vi "Lab Panel V5.22.1.vi"() -> ()   [LabVIEW 2013] (continued)
                            n2498 = Bundle(cluster=w4642, "amps"=w4646, "volts"=w4645, "pf"=w4644) -> (w4643:cluster{"amps":dbl, "volts":dbl, "pf":dbl})
                            n2499 = local write "ON L05-2"(w4643) -> ()
                          }
                        }
                      }
                      frame #1 {
                        n2500 = Unbundle(w4651) -> ("amps"=w4650:dbl, "volts"=w4649:dbl, "pf"=w4648:dbl)
                        n2501 = case shown="True" w4652 {
                          tunnel: w4659 -> [_ w4691]
                          tunnel: w4658 -> [_ w4698]
                          tunnel: w4657 -> [_ _]
                          tunnel: w4656 -> [_ _]
                          tunnel: w4655 -> [_ w4697]
                          tunnel: w4654 -> [_ w4696]
                          tunnel: w4653 -> [_ w4661]
                          tunnel: w4650 -> [_ w4693]
                          tunnel: w4649 -> [_ w4692]
                          tunnel: w4648 -> [_ w4690]
                          tunnel: w4647 -> [_ w4682]
                          frame False {
                          }
                          frame True {
                            n2502 = local read "TDMS LAB05-2"() -> (w4695:refnum<k34>)
                            n2503 = Build Array(w4692) -> (w4687:dbl[])
                            n2504 = Build Array(w4690) -> (w4686:dbl[])
                            n2505 = Build Array(w4697) -> (w4685:dbl[])
                            n2506 = Build Array(w4698) -> (w4684:dbl[])
                            n2507 = Build Array(w4693) -> (w4689:dbl[])
                            n2508 = Build Array(w4691) -> (w4688:dbl[])
                            n2509 = Build Array(w4696) -> (w4683:dbl[])
                            n2510 = Build Array("AMPS ON", "AMPS OFF", "VOLTS", "PF", "TEMP Live", "TEMP Neut", "CYCLE") -> (w4666:string[])
                            n2511 = Bundle By Name("Y"=w4689, "t0"=w4682) -> (w4681:waveform(dbl))  [unwired: 1 in]
                            n2512 = Bundle By Name("Y"=w4688, "t0"=w4682) -> (w4680:waveform(dbl))  [unwired: 1 in]
                            n2513 = Bundle By Name("Y"=w4687, "t0"=w4682) -> (w4679:waveform(dbl))  [unwired: 1 in]
                            n2514 = Bundle By Name("Y"=w4686, "t0"=w4682) -> (w4678:waveform(dbl))  [unwired: 1 in]
                            n2515 = Bundle By Name("Y"=w4685, "t0"=w4682) -> (w4677:waveform(dbl))  [unwired: 1 in]
                            n2516 = Bundle By Name("Y"=w4684, "t0"=w4682) -> (w4676:waveform(dbl))  [unwired: 1 in]
                            n2517 = Bundle By Name("Y"=w4683, "t0"=w4682) -> (w4675:waveform(dbl))  [unwired: 1 in]
                            n2518 = Build Array(w4681, w4680, w4679, w4678, w4677, w4676, w4675) -> (w4674:waveform(dbl)[])
                            n2519 = TDMS Write(0:w4695, 5:"TEST VALUES", 7:w4666, 9:w4674) -> (4:w4665:refnum<k34>, 6:w4664:string, 15:w4663:errorcluster)  [unwired: 2 in, 1 out]
                            n2520 = TDMS Write(0:w4665, 5:w4664, 7:"TIME", 9:w4661, 11:w4663) -> (15:w4660:errorcluster)  [unwired: 1 in, 3 out]
                            n2521 = local write "data file error"(w4660) -> ()
                          }
                        }
                      }
                    }
                  }
                }
              }
            }
          }
          frame #13 {
            # "display test values on chart"
            n2522 = local read "jig cycle"() -> (w4703:dbl)
            n2523 = local read "on loops"() -> (w4705:dbl)
            n2524 = Add(x=w4705, y=2) -> (x+y=w4702:dbl)
            n2525 = Equal?(x=w4703, y=1) -> (x = y?=w4701:bool)
            n2526 = Equal?(x=w4703, y=w4702) -> (x = y?=w4700:bool)
            n2527 = Or(x=w4701, y=w4700) -> (x .or. y?=w4699:bool)
            "graph flag" <- w4699
            n2528 = global write "Global display 3.vi" "graph flag"(w4699) -> ()
            n2529 = case shown="True" w4699 {
              frame False {
              }
              frame True {
                n2530 = local read "SIG LAB05-1"() -> (w4748:T2)
                n2531 = local read "SIG LAB04-2"() -> (w4749:T2)
                n2532 = local read "SIG LAB05-2"() -> (w4747:T2)
                n2533 = local read "SIG LAB04-1"() -> (w4750:T2)
                n2534 = local read "SIG LAB03-1"() -> (w4752:T2)
                n2535 = local read "SIG LAB03-2"() -> (w4751:T2)
                n2536 = local read "SIG LAB01-1"() -> (w4756:T2)
                n2537 = local read "SIG LAB02-2"() -> (w4753:T2)
                n2538 = local read "SIG LAB02-1"() -> (w4754:T2)
                n2539 = local read "SIG LAB01-2"() -> (w4755:T2)
                n2540 = Unbundle(w4749) -> ("AMPS"=w4739:dbl, "VOLTS"=w4729:dbl, "Tmp Live"=w4719:dbl, "Tmp Neut"=w4709:dbl)  [unwired: 1 out]
                n2541 = Unbundle(w4748) -> ("AMPS"=w4738:dbl, "VOLTS"=w4728:dbl, "Tmp Live"=w4718:dbl, "Tmp Neut"=w4708:dbl)  [unwired: 1 out]
                n2542 = Unbundle(w4747) -> ("AMPS"=w4737:dbl, "VOLTS"=w4727:dbl, "Tmp Live"=w4717:dbl, "Tmp Neut"=w4707:dbl)  [unwired: 1 out]
                n2543 = Unbundle(w4750) -> ("AMPS"=w4740:dbl, "VOLTS"=w4730:dbl, "Tmp Live"=w4720:dbl, "Tmp Neut"=w4710:dbl)  [unwired: 1 out]
                n2544 = Unbundle(w4751) -> ("AMPS"=w4741:dbl, "VOLTS"=w4731:dbl, "Tmp Live"=w4721:dbl, "Tmp Neut"=w4711:dbl)  [unwired: 1 out]
                n2545 = Unbundle(w4752) -> ("AMPS"=w4742:dbl, "VOLTS"=w4732:dbl, "Tmp Live"=w4722:dbl, "Tmp Neut"=w4712:dbl)  [unwired: 1 out]
                n2546 = Unbundle(w4753) -> ("AMPS"=w4743:dbl, "VOLTS"=w4733:dbl, "Tmp Live"=w4723:dbl, "Tmp Neut"=w4713:dbl)  [unwired: 1 out]
                n2547 = Unbundle(w4754) -> ("AMPS"=w4744:dbl, "VOLTS"=w4734:dbl, "Tmp Live"=w4724:dbl, "Tmp Neut"=w4714:dbl)  [unwired: 1 out]
                n2548 = Unbundle(w4756) -> ("AMPS"=w4746:dbl, "VOLTS"=w4736:dbl, "Tmp Live"=w4726:dbl, "Tmp Neut"=w4716:dbl)  [unwired: 1 out]
                n2549 = Unbundle(w4755) -> ("AMPS"=w4745:dbl, "VOLTS"=w4735:dbl, "Tmp Live"=w4725:dbl, "Tmp Neut"=w4715:dbl)  [unwired: 1 out]
                n2550 = stacked-sequence {
                  tunnel: w4746 -> [w4788 _ _]
                  tunnel: w4745 -> [w4787 _ _]
                  tunnel: w4744 -> [w4778 _ _]
                  tunnel: w4743 -> [w4777 _ _]
                  tunnel: w4742 -> [w4767 _ _]
                  tunnel: w4741 -> [w4766 _ _]
                  tunnel: w4740 -> [_ w4811 _]
                  tunnel: w4739 -> [_ w4810 _]
                  tunnel: w4738 -> [_ w4800 _]
                  tunnel: w4737 -> [_ w4799 _]
                  tunnel: w4736 -> [w4785 _ _]
                  tunnel: w4735 -> [w4784 _ _]
                  tunnel: w4734 -> [w4775 _ _]
                  tunnel: w4733 -> [w4774 _ _]
                  tunnel: w4732 -> [w4765 _ _]
                  tunnel: w4731 -> [w4764 _ _]
                  tunnel: w4730 -> [_ w4809 _]
                  tunnel: w4729 -> [_ w4808 _]
                  tunnel: w4728 -> [_ w4798 _]
                  tunnel: w4727 -> [_ w4797 _]
                  tunnel: w4726 -> [w4782 _ _]
                  tunnel: w4725 -> [w4780 _ _]
                  tunnel: w4724 -> [w4771 _ _]
                  tunnel: w4723 -> [w4769 _ _]
                  tunnel: w4722 -> [w4763 _ _]
                  tunnel: w4721 -> [w4761 _ _]
                  tunnel: w4720 -> [_ w4807 _]
                  tunnel: w4719 -> [_ w4805 _]
                  tunnel: w4718 -> [_ w4796 _]
                  tunnel: w4717 -> [_ w4794 _]
                  tunnel: w4716 -> [w4781 _ _]
                  tunnel: w4715 -> [w4779 _ _]
                  tunnel: w4714 -> [w4770 _ _]
                  tunnel: w4713 -> [w4768 _ _]
                  tunnel: w4712 -> [w4762 _ _]
                  tunnel: w4711 -> [w4760 _ _]
                  tunnel: w4710 -> [_ w4806 _]
                  tunnel: w4709 -> [_ w4804 _]
                  tunnel: w4708 -> [_ w4795 _]
                  tunnel: w4707 -> [_ w4793 _]
                  frame #0 {
                    n2551 = Merge Signals(w4788, w4787) -> (→"LAB01 AMPS":dynamicdata)
                    n2552 = Merge Signals(w4785, w4784) -> (→"LAB01 VOLTS":dynamicdata)
                    n2553 = Merge Signals(w4765, w4764) -> (→"LAB03 VOLTS":dynamicdata)
                    n2554 = Merge Signals(w4782, w4781, w4780, w4779) -> (→"LAB01 deg C":dynamicdata)
                    n2555 = Merge Signals(w4778, w4777) -> (→"LAB02 AMPS":dynamicdata)
                    n2556 = Merge Signals(w4771, w4770, w4769, w4768) -> (→"LAB02 deg C":dynamicdata)
                    n2557 = Merge Signals(w4763, w4762, w4761, w4760) -> (→"LAB03 deg C":dynamicdata)
                    n2558 = Merge Signals(w4775, w4774) -> (→"LAB02 VOLTS":dynamicdata)
                    n2559 = Merge Signals(w4767, w4766) -> (→"LAB03 AMPS":dynamicdata)
                  }
                  frame #1 {
                    n2560 = Merge Signals(w4798, w4797) -> (→"LAB05 VOLTS":dynamicdata)
                    n2561 = Merge Signals(w4811, w4810) -> (→"LAB04 AMPS":dynamicdata)
                    n2562 = Merge Signals(w4800, w4799) -> (→"LAB05 AMPS":dynamicdata)
                    n2563 = Merge Signals(w4796, w4795, w4794, w4793) -> (→"LAB05 deg C":dynamicdata)
                    n2564 = Merge Signals(w4807, w4806, w4805, w4804) -> (→"LAB04 deg C":dynamicdata)
                    n2565 = Merge Signals(w4809, w4808) -> (→"LAB04 VOLTS":dynamicdata)
                  }
                  frame #2 {
                    n2566 = local read "LAB05 VOLTS"() -> (w4819:dynamicdata)
                    n2567 = local read "LAB04 VOLTS"() -> (w4820:dynamicdata)
                    n2568 = local read "LAB02 VOLTS"() -> (w4822:dynamicdata)
                    n2569 = local read "LAB03 VOLTS"() -> (w4821:dynamicdata)
                    n2570 = local read "LAB05 AMPS"() -> (w4825:dynamicdata)
                    n2571 = local read "LAB01 VOLTS"() -> (w4823:dynamicdata)
                    n2572 = local read "LAB04 AMPS"() -> (w4826:dynamicdata)
                    n2573 = local read "LAB03 AMPS"() -> (w4827:dynamicdata)
                    n2574 = local read "LAB03 deg C"() -> (w4815:dynamicdata)
                    n2575 = local read "LAB02 AMPS"() -> (w4828:dynamicdata)
                    n2576 = local read "LAB04 deg C"() -> (w4814:dynamicdata)
                    n2577 = local read "LAB05 deg C"() -> (w4813:dynamicdata)
                    n2578 = local read "LAB02 deg C"() -> (w4816:dynamicdata)
                    n2579 = local read "LAB01 deg C"() -> (w4817:dynamicdata)
                    n2580 = local read "LAB01 AMPS"() -> (w4829:dynamicdata)
                    n2581 = Merge Signals(w4817, w4816, w4815, w4814, w4813) -> (w4812:dynamicdata)
                    n2582 = Merge Signals(w4829, w4828, w4827, w4826, w4825) -> (w4824:dynamicdata)
                    n2583 = Merge Signals(w4823, w4822, w4821, w4820, w4819) -> (w4818:dynamicdata)
                    n2584 = global write "Global display 3.vi" "graph volts"(w4818) -> ()
                    n2585 = global write "Global display 3.vi" "graph deg C"(w4812) -> ()
                    n2586 = global write "Global display 3.vi" "graph amps"(w4824) -> ()
                  }
                }
              }
            }
          }
          frame #14 {
            # "check for amps fail"
            # "check for cycle test & temperature rise fail conditions"
            n2587 = local read "on loops"() -> (w4856:dbl)
            n2588 = local read "jig cycle"() -> (w4853:dbl)
            n2589 = local read "jig cycle"() -> (w4858:dbl)
            n2590 = Add(x=w4856, y=3.0) -> (x+y=w4854:dbl)
            n2591 = Equal?(x=w4853, y=w4854) -> (x = y?=w4849:bool)
            n2592 = local read "Fail Loops"() -> (w4830:dbl)
            n2593 = Equal?(x=w4858, y=1.0) -> (x = y?=w4851:bool)
            n2594 = global write "Global 1.vi" "fail count"(w4830) -> ()
            n2595 = stacked-sequence {
              tunnel: w4852 -> [w4861 _ _ _ _ _ _ _ _ _]
              tunnel: w4851 -> [w4862 w4882 w4902 w4922 w4942 w4962 w4982 w5002 w5022 w5042]
              tunnel: w4850 -> [w4859 _ _ _ _ _ _ _ _ _]
              tunnel: w4849 -> [w4860 w4881 w4901 w4921 w4941 w4961 w4981 w5001 w5021 w5041]
              tunnel: w4848 -> [_ w4880 _ _ _ _ _ _ _ _]
              tunnel: w4847 -> [_ w4879 _ _ _ _ _ _ _ _]
              tunnel: w4846 -> [_ _ w4900 _ _ _ _ _ _ _]
              tunnel: w4845 -> [_ _ w4899 _ _ _ _ _ _ _]
              tunnel: w4844 -> [_ _ _ w4920 _ _ _ _ _ _]
              tunnel: w4843 -> [_ _ _ w4919 _ _ _ _ _ _]
              tunnel: w4842 -> [_ _ _ _ w4940 _ _ _ _ _]
              tunnel: w4841 -> [_ _ _ _ w4939 _ _ _ _ _]
              tunnel: w4840 -> [_ _ _ _ _ w4960 _ _ _ _]
              tunnel: w4839 -> [_ _ _ _ _ w4959 _ _ _ _]
              tunnel: w4838 -> [_ _ _ _ _ _ w4980 _ _ _]
              tunnel: w4837 -> [_ _ _ _ _ _ w4979 _ _ _]
              tunnel: w4836 -> [_ _ _ _ _ _ _ w5000 _ _]
              tunnel: w4835 -> [_ _ _ _ _ _ _ w4999 _ _]
              tunnel: w4834 -> [_ _ _ _ _ _ _ _ w5020 _]
              tunnel: w4833 -> [_ _ _ _ _ _ _ _ w5019 _]
              tunnel: w4832 -> [_ _ _ _ _ _ _ _ _ w5040]
              tunnel: w4831 -> [_ _ _ _ _ _ _ _ _ w5039]
              frame #0 {
                # "LAB01-1"
                n2596 = case shown="True" w4859 {
                  tunnel: w4862 -> [_ w4875]
                  tunnel: w4861 -> [_ w4872]
                  tunnel: w4860 -> [_ w4871]
                  frame False {
                  }
                  frame True {
                    n2597 = local read "TEMP START LAB01-1"() -> (w4877:cluster{"TL":dbl, "TN":dbl})
                    n2598 = local read "RESULT LAB01-1"() -> (w4866:bool)
                    n2599 = local read "FAIL LAB01-1"() -> (w4869:cluster{"LO":dbl, "HI":dbl})
                    n2600 = local read "TDMS LAB01-1"() -> (w4876:refnum<k34>)
                    n2601 = local read "SET LAB01-1"() -> (w4873:T5)
                    n2602 = local read "DISP LAB01-1"() -> (w4874:T4)
                    n2603 = local read "SIG LAB01-1"() -> (w4878:T2)
                    n2604 = Bundle("FAIL LAB01-1"=w4869, "SIG LAB01-1"=w4878, "TEMP START LAB01-1"=w4877, "DISP LAB01-1"=w4874, "SET LAB01-1"=w4873, "TDMS LAB01-1"=w4876) -> (w4863:T33)  [unwired: 1 in]
                    n2605 = call "sub vi - cycle&temp fail v7.vi"("Amps Lo?"=w4875, "Input Cluster"=w4863, "SELECT"=w4872, "Amps Hi?"=w4871, "Result In"=w4866) -> ("(FAIL) out"=w4868:cluster{"FAIL LO":dbl, "FAIL HI":dbl}, "(DISP) out"=w4864:T4, "T-RISE"=w4865:cluster{"T-RISE (L)":dbl, "T-RISE (N)":dbl}, "Result Out"=w4867:bool, "file error"=w4870:errorcluster)  [unwired: 10 in]
                    n2606 = local write "TEMP RISE LAB01-1"(w4865) -> ()
                    n2607 = local write "FAIL LAB01-1"(w4868) -> ()
                    n2608 = local write "DISP LAB01-1"(w4864) -> ()
                    n2609 = local write "RESULT LAB01-1"(w4867) -> ()
                    n2610 = local write "data file error"(w4870) -> ()
                  }
                }
              }
              frame #1 {
                # "LAB01-2"
                n2611 = case shown="True" w4880 {
                  tunnel: w4882 -> [_ w4895]
                  tunnel: w4879 -> [_ w4892]
                  tunnel: w4881 -> [_ w4891]
                  frame False {
                  }
                  frame True {
                    n2612 = local read "TEMP START LAB01-2"() -> (w4897:cluster{"TL":dbl, "TN":dbl})
                    n2613 = local read "FAIL LAB01-2"() -> (w4888:cluster{"LO":dbl, "HI":dbl})
                    n2614 = local read "TDMS LAB01-2"() -> (w4896:refnum<k34>)
                    n2615 = local read "SET LAB01-2"() -> (w4893:T5)
                    n2616 = local read "DISP LAB01-2"() -> (w4894:T4)
                    n2617 = local read "RESULT LAB01-2"() -> (w4885:bool)
                    n2618 = local read "SIG LAB01-2"() -> (w4898:T2)
                    n2619 = Bundle("FAIL LAB01-2"=w4888, "SIG LAB01-2"=w4898, "TEMP START LAB01-2"=w4897, "DISP LAB01-2"=w4894, "SET LAB01-2"=w4893, "TDMS LAB01-2"=w4896) -> (w4883:T34)  [unwired: 1 in]
                    n2620 = call "sub vi - cycle&temp fail v7.vi"("Amps Lo?"=w4895, "Input Cluster"=w4883, "SELECT"=w4892, "Amps Hi?"=w4891, "Result In"=w4885) -> ("(FAIL) out"=w4887:cluster{"FAIL LO":dbl, "FAIL HI":dbl}, "(DISP) out"=w4890:T4, "T-RISE"=w4884:cluster{"T-RISE (L)":dbl, "T-RISE (N)":dbl}, "Result Out"=w4886:bool, "file error"=w4889:errorcluster)  [unwired: 10 in]
                    n2621 = local write "TEMP RISE LAB01-2"(w4884) -> ()
                    n2622 = local write "FAIL LAB01-2"(w4887) -> ()
                    n2623 = local write "DISP LAB01-2"(w4890) -> ()
                    n2624 = local write "RESULT LAB01-2"(w4886) -> ()
                    n2625 = local write "data file error"(w4889) -> ()
                  }
                }
              }
              frame #2 {
                # "LAB02-1"
                n2626 = case shown="True" w4900 {
                  tunnel: w4902 -> [_ w4915]
                  tunnel: w4899 -> [_ w4912]
                  tunnel: w4901 -> [_ w4911]
                  frame False {
                  }
                  frame True {
                    n2627 = local read "TEMP START LAB02-1"() -> (w4917:cluster{"TL":dbl, "TN":dbl})
                    n2628 = local read "FAIL LAB02-1"() -> (w4908:cluster{"LO":dbl, "HI":dbl})
                    n2629 = local read "TDMS LAB02-1"() -> (w4916:refnum<k34>)
                    n2630 = local read "SET LAB02-1"() -> (w4913:T5)
                    n2631 = local read "DISP LAB02-1"() -> (w4914:T4)
                    n2632 = local read "SIG LAB02-1"() -> (w4918:T2)
                    n2633 = local read "RESULT LAB02-1"() -> (w4905:bool)
                    n2634 = Bundle("FAIL LAB02-1"=w4908, "SIG LAB02-1"=w4918, "TEMP START LAB02-1"=w4917, "DISP LAB02-1"=w4914, "SET LAB02-1"=w4913, "TDMS LAB02-1"=w4916) -> (w4903:T35)  [unwired: 1 in]
                    n2635 = call "sub vi - cycle&temp fail v7.vi"("Amps Lo?"=w4915, "Input Cluster"=w4903, "SELECT"=w4912, "Amps Hi?"=w4911, "Result In"=w4905) -> ("(FAIL) out"=w4907:cluster{"FAIL LO":dbl, "FAIL HI":dbl}, "(DISP) out"=w4910:T4, "T-RISE"=w4904:cluster{"T-RISE (L)":dbl, "T-RISE (N)":dbl}, "Result Out"=w4906:bool, "file error"=w4909:errorcluster)  [unwired: 10 in]
                    n2636 = local write "TEMP RISE LAB02-1"(w4904) -> ()
                    n2637 = local write "FAIL LAB02-1"(w4907) -> ()
                    n2638 = local write "DISP LAB02-1"(w4910) -> ()
                    n2639 = local write "RESULT LAB02-1"(w4906) -> ()
                    n2640 = local write "data file error"(w4909) -> ()
                  }
                }
              }
              frame #3 {
                # "LAB02-2"
                n2641 = case shown="True" w4920 {
                  tunnel: w4922 -> [_ w4935]
                  tunnel: w4919 -> [_ w4932]
                  tunnel: w4921 -> [_ w4931]
                  frame False {
                  }
                  frame True {
                    n2642 = local read "TEMP START LAB02-2"() -> (w4937:cluster{"TL":dbl, "TN":dbl})
                    n2643 = local read "FAIL LAB02-2"() -> (w4928:cluster{"LO":dbl, "HI":dbl})
                    n2644 = local read "TDMS LAB02-2"() -> (w4936:refnum<k34>)
                    n2645 = local read "SET LAB02-2"() -> (w4933:T5)
                    n2646 = local read "DISP LAB02-2"() -> (w4934:T4)
                    n2647 = local read "SIG LAB02-2"() -> (w4938:T2)
                    n2648 = local read "RESULT LAB02-2"() -> (w4925:bool)
                    n2649 = Bundle("FAIL LAB02-2"=w4928, "SIG LAB02-2"=w4938, "TEMP START LAB02-2"=w4937, "DISP LAB02-2"=w4934, "SET LAB02-2"=w4933, "TDMS LAB02-2"=w4936) -> (w4923:T36)  [unwired: 1 in]
                    n2650 = call "sub vi - cycle&temp fail v7.vi"("Amps Lo?"=w4935, "Input Cluster"=w4923, "SELECT"=w4932, "Amps Hi?"=w4931, "Result In"=w4925) -> ("(FAIL) out"=w4927:cluster{"FAIL LO":dbl, "FAIL HI":dbl}, "(DISP) out"=w4930:T4, "T-RISE"=w4924:cluster{"T-RISE (L)":dbl, "T-RISE (N)":dbl}, "Result Out"=w4926:bool, "file error"=w4929:errorcluster)  [unwired: 10 in]
                    n2651 = local write "TEMP RISE LAB02-2"(w4924) -> ()
                    n2652 = local write "FAIL LAB02-2"(w4927) -> ()
                    n2653 = local write "DISP LAB02-2"(w4930) -> ()
                    n2654 = local write "RESULT LAB02-2"(w4926) -> ()
                    n2655 = local write "data file error"(w4929) -> ()
                  }
                }
              }
              frame #4 {
                # "LAB03-1"
                n2656 = case shown="True" w4940 {
                  tunnel: w4942 -> [_ w4955]
                  tunnel: w4939 -> [_ w4952]
                  tunnel: w4941 -> [_ w4951]
                  frame False {
                  }
                  frame True {
                    n2657 = local read "TEMP START LAB03-1"() -> (w4957:cluster{"TL":dbl, "TN":dbl})
                    n2658 = local read "FAIL LAB03-1"() -> (w4948:cluster{"LO":dbl, "HI":dbl})
                    n2659 = local read "TDMS LAB03-1"() -> (w4956:refnum<k34>)
                    n2660 = local read "SET LAB03-1"() -> (w4953:T5)
                    n2661 = local read "DISP LAB03-1"() -> (w4954:T4)
                    n2662 = local read "SIG LAB03-1"() -> (w4958:T2)
                    n2663 = local read "RESULT LAB03-1"() -> (w4945:bool)
                    n2664 = Bundle("FAIL LAB03-1"=w4948, "SIG LAB03-1"=w4958, "TEMP START LAB03-1"=w4957, "DISP LAB03-1"=w4954, "SET LAB03-1"=w4953, "TDMS LAB03-1"=w4956) -> (w4943:T37)  [unwired: 1 in]
                    n2665 = call "sub vi - cycle&temp fail v7.vi"("Amps Lo?"=w4955, "Input Cluster"=w4943, "SELECT"=w4952, "Amps Hi?"=w4951, "Result In"=w4945) -> ("(FAIL) out"=w4947:cluster{"FAIL LO":dbl, "FAIL HI":dbl}, "(DISP) out"=w4950:T4, "T-RISE"=w4944:cluster{"T-RISE (L)":dbl, "T-RISE (N)":dbl}, "Result Out"=w4946:bool, "file error"=w4949:errorcluster)  [unwired: 10 in]
                    n2666 = local write "TEMP RISE LAB03-1"(w4944) -> ()
                    n2667 = local write "FAIL LAB03-1"(w4947) -> ()
                    n2668 = local write "DISP LAB03-1"(w4950) -> ()
                    n2669 = local write "RESULT LAB03-1"(w4946) -> ()
                    n2670 = local write "data file error"(w4949) -> ()
                  }
                }
              }
              frame #5 {
                # "LAB03-2"
                n2671 = case shown="True" w4960 {
                  tunnel: w4962 -> [_ w4975]
                  tunnel: w4959 -> [_ w4972]
                  tunnel: w4961 -> [_ w4971]
                  frame False {
                  }
                  frame True {
                    n2672 = local read "TEMP START LAB03-2"() -> (w4977:cluster{"TL":dbl, "TN":dbl})
                    n2673 = local read "FAIL LAB03-2"() -> (w4968:cluster{"LO":dbl, "HI":dbl})
                    n2674 = local read "TDMS LAB03-2"() -> (w4976:refnum<k34>)
                    n2675 = local read "SET LAB03-2"() -> (w4973:T5)
                    n2676 = local read "DISP LAB03-2"() -> (w4974:T4)
                    n2677 = local read "RESULT LAB03-2"() -> (w4965:bool)
                    n2678 = local read "SIG LAB03-2"() -> (w4978:T2)
                    n2679 = Bundle("FAIL LAB03-2"=w4968, "SIG LAB03-2"=w4978, "TEMP START LAB03-2"=w4977, "DISP LAB03-2"=w4974, "SET LAB03-2"=w4973, "TDMS LAB03-2"=w4976) -> (w4963:T38)  [unwired: 1 in]
                    n2680 = call "sub vi - cycle&temp fail v7.vi"("Amps Lo?"=w4975, "Input Cluster"=w4963, "SELECT"=w4972, "Amps Hi?"=w4971, "Result In"=w4965) -> ("(FAIL) out"=w4967:cluster{"FAIL LO":dbl, "FAIL HI":dbl}, "(DISP) out"=w4970:T4, "T-RISE"=w4964:cluster{"T-RISE (L)":dbl, "T-RISE (N)":dbl}, "Result Out"=w4966:bool, "file error"=w4969:errorcluster)  [unwired: 10 in]
                    n2681 = local write "FAIL LAB03-2"(w4967) -> ()
                    n2682 = local write "TEMP RISE LAB03-2"(w4964) -> ()
                    n2683 = local write "DISP LAB03-2"(w4970) -> ()
                    n2684 = local write "RESULT LAB03-2"(w4966) -> ()
                    n2685 = local write "data file error"(w4969) -> ()
                  }
                }
              }
              frame #6 {
                # "LAB04-1"
                n2686 = case shown="True" w4980 {
                  tunnel: w4982 -> [_ w4995]
                  tunnel: w4979 -> [_ w4992]
                  tunnel: w4981 -> [_ w4991]
                  frame False {
                  }
                  frame True {
                    n2687 = local read "TEMP START LAB04-1"() -> (w4997:cluster{"TL":dbl, "TN":dbl})
                    n2688 = local read "FAIL LAB04-1"() -> (w4988:cluster{"LO":dbl, "HI":dbl})
                    n2689 = local read "TDMS LAB04-1"() -> (w4996:refnum<k34>)
                    n2690 = local read "SET LAB04-1"() -> (w4993:T5)
                    n2691 = local read "DISP LAB04-1"() -> (w4994:T4)
                    n2692 = local read "SIG LAB04-1"() -> (w4998:T2)
                    n2693 = local read "RESULT LAB04-1"() -> (w4985:bool)
                    n2694 = Bundle("FAIL LAB04-1"=w4988, "SIG LAB04-1"=w4998, "TEMP START LAB04-1"=w4997, "DISP LAB04-1"=w4994, "SET LAB04-1"=w4993, "TDMS LAB04-1"=w4996) -> (w4983:T39)  [unwired: 1 in]
                    n2695 = call "sub vi - cycle&temp fail v7.vi"("Amps Lo?"=w4995, "Input Cluster"=w4983, "SELECT"=w4992, "Amps Hi?"=w4991, "Result In"=w4985) -> ("(FAIL) out"=w4987:cluster{"FAIL LO":dbl, "FAIL HI":dbl}, "(DISP) out"=w4990:T4, "T-RISE"=w4984:cluster{"T-RISE (L)":dbl, "T-RISE (N)":dbl}, "Result Out"=w4986:bool, "file error"=w4989:errorcluster)  [unwired: 10 in]
                    n2696 = local write "TEMP RISE LAB04-1"(w4984) -> ()
                    n2697 = local write "FAIL LAB04-1"(w4987) -> ()
                    n2698 = local write "DISP LAB04-1"(w4990) -> ()
                    n2699 = local write "RESULT LAB04-1"(w4986) -> ()
                    n2700 = local write "data file error"(w4989) -> ()
                  }
                }
              }
              frame #7 {
                # "LAB04-2"
                n2701 = case shown="True" w5000 {
                  tunnel: w5002 -> [_ w5015]
                  tunnel: w4999 -> [_ w5012]
                  tunnel: w5001 -> [_ w5011]
                  frame False {
                  }
                  frame True {
                    n2702 = local read "TEMP START LAB04-2"() -> (w5017:cluster{"TL":dbl, "TN":dbl})
                    n2703 = local read "FAIL LAB04-2"() -> (w5008:cluster{"LO":dbl, "HI":dbl})
                    n2704 = local read "TDMS LAB04-2"() -> (w5016:refnum<k34>)
                    n2705 = local read "SET LAB04-2"() -> (w5013:T5)
                    n2706 = local read "DISP LAB04-2"() -> (w5014:T4)
                    n2707 = local read "SIG LAB04-2"() -> (w5018:T2)
                    n2708 = local read "RESULT LAB04-2"() -> (w5005:bool)
                    n2709 = Bundle("FAIL LAB04-2"=w5008, "SIG LAB04-2"=w5018, "TEMP START LAB04-2"=w5017, "DISP LAB04-2"=w5014, "SET LAB04-2"=w5013, "TDMS LAB04-2"=w5016) -> (w5003:T40)  [unwired: 1 in]
                    n2710 = call "sub vi - cycle&temp fail v7.vi"("Amps Lo?"=w5015, "Input Cluster"=w5003, "SELECT"=w5012, "Amps Hi?"=w5011, "Result In"=w5005) -> ("(FAIL) out"=w5007:cluster{"FAIL LO":dbl, "FAIL HI":dbl}, "(DISP) out"=w5010:T4, "T-RISE"=w5004:cluster{"T-RISE (L)":dbl, "T-RISE (N)":dbl}, "Result Out"=w5006:bool, "file error"=w5009:errorcluster)  [unwired: 10 in]
                    n2711 = local write "TEMP RISE LAB04-2"(w5004) -> ()
                    n2712 = local write "FAIL LAB04-2"(w5007) -> ()
                    n2713 = local write "DISP LAB04-2"(w5010) -> ()
                    n2714 = local write "RESULT LAB04-2"(w5006) -> ()
                    n2715 = local write "data file error"(w5009) -> ()
                  }
                }
              }
              frame #8 {
                # "LAB05-1"
                n2716 = case shown="True" w5020 {
                  tunnel: w5022 -> [_ w5035]
                  tunnel: w5019 -> [_ w5032]
                  tunnel: w5021 -> [_ w5031]
                  frame False {
                  }
                  frame True {
                    n2717 = local read "TEMP START LAB05-1"() -> (w5037:cluster{"TL":dbl, "TN":dbl})
                    n2718 = local read "FAIL LAB05-1"() -> (w5028:cluster{"LO":dbl, "HI":dbl})
                    n2719 = local read "TDMS LAB05-1"() -> (w5036:refnum<k34>)
                    n2720 = local read "SET LAB05-1"() -> (w5033:T5)
                    n2721 = local read "DISP LAB05-1"() -> (w5034:T4)
                    n2722 = local read "SIG LAB05-1"() -> (w5038:T2)
                    n2723 = local read "RESULT LAB05-1"() -> (w5025:bool)
                    n2724 = Bundle("FAIL LAB05-1"=w5028, "SIG LAB05-1"=w5038, "TEMP START LAB05-1"=w5037, "DISP LAB05-1"=w5034, "SET LAB05-1"=w5033, "TDMS LAB05-1"=w5036) -> (w5023:T41)  [unwired: 1 in]
                    n2725 = call "sub vi - cycle&temp fail v7.vi"("Amps Lo?"=w5035, "Input Cluster"=w5023, "SELECT"=w5032, "Amps Hi?"=w5031, "Result In"=w5025) -> ("(FAIL) out"=w5027:cluster{"FAIL LO":dbl, "FAIL HI":dbl}, "(DISP) out"=w5030:T4, "T-RISE"=w5024:cluster{"T-RISE (L)":dbl, "T-RISE (N)":dbl}, "Result Out"=w5026:bool, "file error"=w5029:errorcluster)  [unwired: 10 in]
                    n2726 = local write "TEMP RISE LAB05-1"(w5024) -> ()
                    n2727 = local write "FAIL LAB05-1"(w5027) -> ()
                    n2728 = local write "DISP LAB05-1"(w5030) -> ()
                    n2729 = local write "RESULT LAB05-1"(w5026) -> ()
                    n2730 = local write "data file error"(w5029) -> ()
                  }
                }
              }
              frame #9 {
                # "LAB05-2"
                n2731 = case shown="True" w5040 {
                  tunnel: w5042 -> [_ w5055]
                  tunnel: w5039 -> [_ w5052]
                  tunnel: w5041 -> [_ w5051]
                  frame False {
                  }
                  frame True {
                    n2732 = local read "TEMP START LAB05-2"() -> (w5057:cluster{"TL":dbl, "TN":dbl})
                    n2733 = local read "FAIL LAB05-2"() -> (w5048:cluster{"LO":dbl, "HI":dbl})
                    n2734 = local read "TDMS LAB05-2"() -> (w5056:refnum<k34>)
                    n2735 = local read "SET LAB05-2"() -> (w5053:T5)
                    n2736 = local read "DISP LAB05-2"() -> (w5054:T4)
                    n2737 = local read "SIG LAB05-2"() -> (w5058:T2)
                    n2738 = local read "RESULT LAB05-2"() -> (w5045:bool)
                    n2739 = Bundle("FAIL LAB05-2"=w5048, "SIG LAB05-2"=w5058, "TEMP START LAB05-2"=w5057, "DISP LAB05-2"=w5054, "SET LAB05-2"=w5053, "TDMS LAB05-2"=w5056) -> (w5043:T42)  [unwired: 1 in]
                    n2740 = call "sub vi - cycle&temp fail v7.vi"("Amps Lo?"=w5055, "Input Cluster"=w5043, "SELECT"=w5052, "Amps Hi?"=w5051, "Result In"=w5045) -> ("(FAIL) out"=w5047:cluster{"FAIL LO":dbl, "FAIL HI":dbl}, "(DISP) out"=w5050:T4, "T-RISE"=w5044:cluster{"T-RISE (L)":dbl, "T-RISE (N)":dbl}, "Result Out"=w5046:bool, "file error"=w5049:errorcluster)  [unwired: 10 in]
                    n2741 = local write "TEMP RISE LAB05-2"(w5044) -> ()
                    n2742 = local write "FAIL LAB05-2"(w5047) -> ()
                    n2743 = local write "DISP LAB05-2"(w5050) -> ()
                    n2744 = local write "RESULT LAB05-2"(w5046) -> ()
                    n2745 = local write "data file error"(w5049) -> ()
                  }
                }
              }
            }
          }
          frame #15 {
            # "run calibration routine"
            n2746 = local read "SET (cal)"() -> (w5059:bool)
            n2747 = case shown="True" w5059 {
              frame False {
              }
              frame True {
                n2748 = stacked-sequence {
                  seq-local: [w5060 _ _] -> [_ w5062 _]
                  frame #0 {
                    n2749 = call "CALIBRATION PASSWORD"() -> ("PASSWORD"=w5060:string)  [unwired: 17 in, 2 out]
                  }
                  frame #1 {
                    n2750 = Equal?(x=w5062, y="7777") -> (x = y?=w5061:bool)
                    n2751 = case shown="True" w5061 {
                      frame False {
                      }
                      frame True {
                        n2752 = stacked-sequence {
                          frame #0 {
                            n2753 = local read "Temp Test Cal"() -> (w5064:dbl)
                            n2754 = call "sub vi - calibration v1.vi"("Temp Test Cal"=w5064) -> ()  [unwired: 11 in]
                          }
                          frame #1 {
                            n2755 = call "sub vi - get calibration values v1.vi"() -> ("TEMP REF CAL"=w5065:dbl, "LAB01 (CAL)"=w5070:T14, "LAB02 (CAL)"=w5069:T15, "LAB03 (CAL)"=w5068:T14, "LAB04 (CAL)"=w5067:T14, "calibration file error out"=w5071:errorcluster, "LAB05 (CAL)"=w5066:T14)  [unwired: 9 in]
                            n2756 = local write "TEMP REF cal"(w5065) -> ()
                            n2757 = local write "cal file error out"(w5071) -> ()
                            n2758 = local write "CAL LAB04"(w5067) -> ()
                            n2759 = local write "CAL LAB05"(w5066) -> ()
                            n2760 = local write "CAL LAB01"(w5070) -> ()
                            n2761 = local write "CAL LAB02"(w5069) -> ()
                            n2762 = local write "CAL LAB03"(w5068) -> ()
                          }
                        }
                      }
                    }
                  }
                  frame #2 {
                    n2763 = local write "SET (cal)"(FALSE) -> ()
                  }
                }
              }
            }
          }
          frame #16 {
            # "save certain settings to file"
            n2764 = String To Path(string="c:\\crabtree\\Set Up\\") -> (path=w5074:path)
            n2765 = Build Path(base path=w5074, name or relative path="settings.bin") -> (appended path=w5076:path)
            n2766 = Build Path(base path=w5074, name or relative path="mail.bin") -> (appended path=w5073:path)
            n2767 = Create Folder(path (use dialog)=w5074) -> (error out=w5079:errorcluster)  [unwired: 2 in, 2 out]
            n2768 = call <vilib>:"Clear Errors.vi"("error in (no error)"=w5079) -> ()  [unwired: 6 in, 1 out]
            n2769 = stacked-sequence {
              seq-local: [w5091 _] -> [_ w5104]
              tunnel: w5076 -> [_ w5105]
              tunnel: w5073 -> [_ w5103]
              frame #0 {
                n2770 = local read "C drive data root dir"() -> (w5090:path)
                n2771 = local read "Select COM port"() -> (w5087:refnum<visa-resource-name>)
                n2772 = local read "Network Directory"() -> (w5096:path)
                n2773 = local read "SET LAB05-2"() -> (w5095:T5)
                n2774 = local read "SET LAB05-1"() -> (w5094:T5)
                n2775 = local read "SET LAB04-2"() -> (w5093:T5)
                n2776 = local read "SET LAB03-2"() -> (w5097:T5)
                n2777 = local read "SET LAB04-1"() -> (w5092:T5)
                n2778 = local read "SET LAB03-1"() -> (w5098:T5)
                n2779 = local read "SET LAB02-2"() -> (w5099:T5)
                n2780 = local read "SET LAB02-1"() -> (w5100:T5)
                n2781 = local read "Temp Delay Lps"() -> (w5086:dbl)
                n2782 = local read "Amps Fail level"() -> (w5082:dbl)
                n2783 = local read "SET LAB01-2"() -> (w5101:T5)
                n2784 = local read "Temp Test Cal"() -> (w5083:dbl)
                n2785 = local read "SET LAB01-1"() -> (w5102:T5)
                n2786 = local read "Mail Test File To:"() -> (w5081:string)
                n2787 = local read "Temp Value"() -> (w5085:dbl)
                n2788 = local read "Fail Loops"() -> (w5084:dbl)
                n2789 = local read "Mail Test Fail"() -> (w5080:bool)
                n2790 = local read "RATE (Hz)"() -> (w5089:dbl)
                n2791 = local read "SAMPLES"() -> (w5088:dbl)
                n2792 = Bundle("SET LAB01-1"=w5102, "SET LAB01-2"=w5101, "SET LAB02-1"=w5100, "SET LAB02-2"=w5099, "SET LAB03-1"=w5098, "SET LAB03-2"=w5097, "SET LAB04-1"=w5092, "SET LAB04-2"=w5093, "SET LAB05-1"=w5094, "SET LAB05-2"=w5095, "Network Directory"=w5096, "C drive data root dir"=w5090, "RATE (Hz)"=w5089, "SAMPLES"=w5088, "Select COM port"=w5087, "Temp Delay Lps"=w5086, "Temp Value"=w5085, "Fail Loops"=w5084, "Temp Test Cal"=w5083, "Amps Fail level"=w5082, "Mail Test File To:"=w5081, "Mail Test Fail"=w5080) -> (w5091:T22)  [unwired: 1 in]
              }
              frame #1 {
                n2793 = event shown="[1] \"SET LAB01-1\", \"SET LAB01-2\", \"SET LAB02-1\", \"SET LAB02-2\", \"SET LAB03-1\", \"SET LAB03-2\", \"SET LAB04-1\", \"SET LAB04-2\", \"SET LAB05-1\", \"SET LAB05-2\", \"Network Directory\", \"C drive data root dir\", \"RATE (Hz)\", \"SAMPLES\", \"Select COM port\", \"Temp Delay Lps\", \"Temp Value\", \"Fail Loops\", \"Temp Test Cal\", \"Amps Fail level\", \"Mail Test File To:\", \"Mail Test Fail\": Value Change" {
                  selector: _ -> [_ _ _]
                  dyn-events: _ -> [_ _ _]
                  timeout: 10.0 -> [_ _ _]
                  tunnel: w5105 -> [_ w5107 _]
                  tunnel: w5104 -> [_ w5108 _]
                  tunnel: w5103 -> [_ _ w5119]
                  event Timeout {
                    n2794 = event-data() -> ()  [unwired: 1 in, 3 out]
                  }
                  event "SET LAB01-1", "SET LAB01-2", "SET LAB02-1", "SET LAB02-2", "SET LAB03-1", "SET LAB03-2", "SET LAB04-1", "SET LAB04-2", "SET LAB05-1", "SET LAB05-2", "Network Directory", "C drive data root dir", "RATE (Hz)", "SAMPLES", "Select COM port", "Temp Delay Lps", "Temp Value", "Fail Loops", "Temp Test Cal", "Amps Fail level", "Mail Test File To:", "Mail Test Fail": Value Change {
                    n2795 = event-data() -> ()  [unwired: 1 in, 6 out]
                    n2796 = Open/Create/Replace File(file path (use dialog)=w5107, operation (0:open)=T17."replace or create") -> (refnum out=w5113:refnum<file>, error out=w5112:errorcluster)  [unwired: 4 in, 1 out]
                    n2797 = Write to Binary File(file (use dialog)=w5113, data=w5108, error in=w5112) -> (refnum out=w5111:refnum<file>, error out=w5110:errorcluster)  [unwired: 3 in, 1 out]
                    n2798 = Close File(refnum=w5111, error in=w5110) -> (error out=w5109:errorcluster)  [unwired: 1 out]
                    n2799 = local write "data file error"(w5109) -> ()
                  }
                  event "MAIL SETTINGS.OUT SERVER ADDRESS", "MAIL SETTINGS.FROM ACCOUNT", "MAIL SETTINGS.USER NAME", "MAIL SETTINGS.PASSWORD", "Auto Mail Send", "TO (string):": Value Change {
                    n2800 = event-data() -> ()  [unwired: 1 in, 6 out]
                    n2801 = local read "MAIL SETTINGS"() -> (w5118:T7)
                    n2802 = local read "Auto Mail Send"() -> (w5116:bool)
                    n2803 = local read "TO (string):"() -> (w5115:string)
                    n2804 = Open/Create/Replace File(file path (use dialog)=w5119, operation (0:open)=T17."replace or create") -> (refnum out=w5124:refnum<file>, error out=w5123:errorcluster)  [unwired: 4 in, 1 out]
                    n2805 = Bundle("MAIL SETTINGS"=w5118, "Auto Mail Send"=w5116, "TO (string):"=w5115) -> (w5117:T43)  [unwired: 1 in]
                    n2806 = Write to Binary File(file (use dialog)=w5124, data=w5117, error in=w5123) -> (refnum out=w5122:refnum<file>, error out=w5121:errorcluster)  [unwired: 3 in, 1 out]
                    n2807 = Close File(refnum=w5122, error in=w5121) -> (error out=w5120:errorcluster)  [unwired: 1 out]
                    n2808 = local write "data file error"(w5120) -> ()
                  }
                }
              }
            }
          }
          frame #17 {
            # "mail control"
            n2809 = local read "MAIL SETTINGS"() -> (w5141:T7)
            n2810 = local read "Auto Mail Send"() -> (w5127:bool)
            n2811 = Unbundle(w5141) -> ("OUT SERVER ADDRESS"=w5140:string, "FROM ACCOUNT"=w5139:string, "TEST MAIL"=w5138:bool)  [unwired: 4 out]
            n2812 = stacked-sequence {
              tunnel: "TO (string):" -> [_ w5180]
              tunnel: w5141 -> [w5146 w5179]
              tunnel: w5140 -> [w5145 w5178]
              tunnel: w5139 -> [w5144 w5177]
              tunnel: w5138 -> [w5143 _]
              tunnel: w5127 -> [_ w5176]
              tunnel: w5137 -> [_ w5175]
              tunnel: w5136 -> [_ w5174]
              tunnel: w5135 -> [_ w5173]
              tunnel: w5134 -> [_ w5172]
              tunnel: w5133 -> [_ w5171]
              tunnel: w5132 -> [_ w5170]
              tunnel: w5131 -> [_ w5169]
              tunnel: w5130 -> [_ w5168]
              tunnel: w5129 -> [_ w5167]
              tunnel: w5128 -> [_ w5166]
              tunnel: "TO (string):" -> [w5142 _]
              frame #0 {
                # "mail test"
                n2813 = case shown="True" w5143 {
                  tunnel: w5146 -> [_ w5150]
                  tunnel: w5142 -> [_ w5149]
                  tunnel: w5145 -> [_ w5148]
                  tunnel: w5144 -> [_ w5147]
                  frame False {
                  }
                  frame True {
                    n2814 = stacked-sequence {
                      seq-local: [_ _ w5160 _] -> [_ _ _ w5161]
                      tunnel: w5150 -> [w5153 _ _ w5165]
                      tunnel: w5149 -> [_ _ w5158 _]
                      tunnel: w5148 -> [_ _ w5156 _]
                      tunnel: w5147 -> [_ _ w5157 _]
                      frame #0 {
                        n2815 = Bundle(cluster=w5153, "TEST MAIL STATUS"="TEST START") -> (w5151:T7)  [unwired: 6 in]
                        n2816 = local write "MAIL SETTINGS"(w5151) -> ()
                      }
                      frame #1 {
                        n2817 = Wait (ms)(milliseconds to wait=500) -> ()  [unwired: 1 out]
                      }
                      frame #2 {
                        n2818 = call "sub vi - send mail v5.vi"("TO:"=w5158, "subject"="MAIL TEST FROM LAB PANEL", "from"=w5157, "out going server"=w5156, "message"="TEST MESSAGE") -> ("error out"=w5160:errorcluster)  [unwired: 10 in]
                      }
                      frame #3 {
                        n2819 = Bundle(cluster=w5165, "TEST MAIL"=FALSE, "TEST MAIL STATUS"="TEST END", "mail error"=w5161) -> (w5163:T7)  [unwired: 4 in]
                        n2820 = local write "MAIL SETTINGS"(w5163) -> ()
                      }
                    }
                  }
                }
              }
              frame #1 {
                # "mail report"
                n2821 = stacked-sequence {
                  seq-local: [_ w5223 _ _] -> [_ _ _ w5413]
                  seq-local: [_ _ w5326 _] -> [_ _ _ w5403]
                  seq-local: [w5190 _ _ _] -> [_ w5240 _ _]
                  seq-local: [w5189 _ _ _] -> [_ w5239 _ _]
                  seq-local: [w5187 _ _ _] -> [_ w5237 _ _]
                  seq-local: [w5188 _ _ _] -> [_ w5238 _ _]
                  seq-local: [w5186 _ _ _] -> [_ w5236 _ _]
                  seq-local: [w5185 _ _ _] -> [_ w5231 _ _]
                  seq-local: [w5184 _ _ _] -> [_ w5232 _ _]
                  seq-local: [w5183 _ _ _] -> [_ w5233 _ _]
                  seq-local: [w5182 _ _ _] -> [_ w5234 _ _]
                  seq-local: [w5181 _ _ _] -> [_ w5235 _ _]
                  tunnel: w5180 -> [_ _ _ w5414]
                  tunnel: w5179 -> [_ _ _ w5397]
                  tunnel: w5178 -> [_ _ _ w5411]
                  tunnel: w5177 -> [_ _ _ w5410]
                  tunnel: w5176 -> [w5221 _ _ w5405]
                  tunnel: w5175 -> [_ _ w5356 _]
                  tunnel: w5174 -> [_ _ w5353 _]
                  tunnel: w5173 -> [_ _ w5352 _]
                  tunnel: w5172 -> [_ _ w5351 _]
                  tunnel: w5171 -> [_ _ w5350 _]
                  tunnel: w5170 -> [_ _ w5349 _]
                  tunnel: w5169 -> [_ _ w5348 _]
                  tunnel: w5168 -> [_ _ w5347 _]
                  tunnel: w5167 -> [_ _ w5346 _]
                  tunnel: w5166 -> [_ _ w5345 _]
                  frame #0 {
                    n2822 = case shown="False" w5221 {
                      frame False {
                        n2823 = local write "mail control"("") -> ()
                      }
                      frame True {
                      }
                    }
                    n2824 = local read "SET LAB01-1"() -> (w5220:T5)
                    n2825 = local read "SET LAB01-2"() -> (w5219:T5)
                    n2826 = local read "SET LAB02-1"() -> (w5218:T5)
                    n2827 = local read "SET LAB02-2"() -> (w5217:T5)
                    n2828 = local read "SET LAB03-1"() -> (w5216:T5)
                    n2829 = local read "SET LAB04-1"() -> (w5214:T5)
                    n2830 = local read "SET LAB05-1"() -> (w5212:T5)
                    n2831 = local read "SET LAB03-2"() -> (w5215:T5)
                    n2832 = local read "SET LAB04-2"() -> (w5213:T5)
                    n2833 = local read "SET LAB05-2"() -> (w5211:T5)
                    n2834 = Unbundle(w5216) -> ("DESCRIPTION"=w5196:string)  [unwired: 4 out]
                    n2835 = Unbundle(w5215) -> ("DESCRIPTION"=w5195:string)  [unwired: 4 out]
                    n2836 = Unbundle(w5214) -> ("DESCRIPTION"=w5194:string)  [unwired: 4 out]
                    n2837 = Unbundle(w5211) -> ("DESCRIPTION"=w5191:string)  [unwired: 4 out]
                    n2838 = Unbundle(w5217) -> ("DESCRIPTION"=w5197:string)  [unwired: 4 out]
                    n2839 = Unbundle(w5213) -> ("DESCRIPTION"=w5193:string)  [unwired: 4 out]
                    n2840 = Unbundle(w5220) -> ("DESCRIPTION"=w5209:string)  [unwired: 4 out]
                    n2841 = Unbundle(w5218) -> ("DESCRIPTION"=w5198:string)  [unwired: 4 out]
                    n2842 = Unbundle(w5212) -> ("DESCRIPTION"=w5192:string)  [unwired: 4 out]
                    n2843 = Unbundle(w5219) -> ("DESCRIPTION"=w5199:string)  [unwired: 4 out]
                    n2844 = Concatenate Strings("[LAB05-2/", w5191) -> (w5181:string)
                    n2845 = Concatenate Strings("[LAB05-1/", w5192) -> (w5182:string)
                    n2846 = Concatenate Strings("[LAB04-2/", w5193) -> (w5183:string)
                    n2847 = Concatenate Strings("[LAB03-2/", w5195) -> (w5185:string)
                    n2848 = Concatenate Strings("[LAB04-1/", w5194) -> (w5184:string)
                    n2849 = Concatenate Strings("[LAB03-1/", w5196) -> (w5186:string)
                    n2850 = Concatenate Strings("[LAB01-2/", w5199) -> (w5189:string)
                    n2851 = Concatenate Strings("[LAB02-2/", w5197) -> (w5187:string)
                    n2852 = Concatenate Strings("[LAB01-1/", w5209) -> (w5190:string)
                    n2853 = Concatenate Strings("[LAB02-1/", w5198) -> (w5188:string)
                  }
                  frame #1 {
                    w5244 = "/"
                    w5245 = 2.0
                    n2854 = local read "DISP LAB01-2"() -> (w5324:T4)
                    n2855 = local read "DISP LAB01-1"() -> (w5325:T4)
                    n2856 = local read "DISP LAB02-1"() -> (w5323:T4)
                    n2857 = local read "DISP LAB03-2"() -> (w5320:T4)
                    n2858 = local read "DISP LAB02-2"() -> (w5322:T4)
                    n2859 = local read "DISP LAB03-1"() -> (w5321:T4)
                    n2860 = local read "DISP LAB04-2"() -> (w5318:T4)
                    n2861 = local read "DISP LAB04-1"() -> (w5319:T4)
                    n2862 = local read "DISP LAB05-1"() -> (w5317:T4)
                    n2863 = local read "DISP LAB05-2"() -> (w5316:T4)
                    n2864 = Unbundle(w5324) -> ("CYCLE"=w5308:dbl, "MINS"=w5307:dbl, "STATUS"=w5304:string)
                    n2865 = Unbundle(w5325) -> ("CYCLE"=w5313:dbl, "MINS"=w5312:dbl, "STATUS"=w5309:string)
                    n2866 = Unbundle(w5323) -> ("CYCLE"=w5301:dbl, "MINS"=w5300:dbl, "STATUS"=w5299:string)
                    n2867 = Unbundle(w5320) -> ("CYCLE"=w5288:dbl, "MINS"=w5287:dbl, "STATUS"=w5284:string)
                    n2868 = Unbundle(w5321) -> ("CYCLE"=w5293:dbl, "MINS"=w5292:dbl, "STATUS"=w5289:string)
                    n2869 = Unbundle(w5322) -> ("CYCLE"=w5298:dbl, "MINS"=w5297:dbl, "STATUS"=w5294:string)
                    n2870 = Unbundle(w5319) -> ("CYCLE"=w5283:dbl, "MINS"=w5282:dbl, "STATUS"=w5279:string)
                    n2871 = Unbundle(w5318) -> ("CYCLE"=w5278:dbl, "MINS"=w5277:dbl, "STATUS"=w5274:string)
                    n2872 = Unbundle(w5317) -> ("CYCLE"=w5273:dbl, "MINS"=w5272:dbl, "STATUS"=w5269:string)
                    n2873 = Unbundle(w5316) -> ("CYCLE"=w5315:dbl, "MINS"=w5314:dbl, "STATUS"=w5266:string)
                    n2874 = Number To Decimal String(number=w5301) -> (decimal integer string=w5303:string)  [unwired: 1 in]
                    n2875 = Number To Decimal String(number=w5298) -> (decimal integer string=w5296:string)  [unwired: 1 in]
                    n2876 = Number To Decimal String(number=w5293) -> (decimal integer string=w5291:string)  [unwired: 1 in]
                    n2877 = Number To Decimal String(number=w5308) -> (decimal integer string=w5306:string)  [unwired: 1 in]
                    n2878 = Number To Decimal String(number=w5288) -> (decimal integer string=w5286:string)  [unwired: 1 in]
                    n2879 = Number To Decimal String(number=w5313) -> (decimal integer string=w5311:string)  [unwired: 1 in]
                    n2880 = Number To Decimal String(number=w5315) -> (decimal integer string=w5268:string)  [unwired: 1 in]
                    n2881 = Number To Decimal String(number=w5283) -> (decimal integer string=w5281:string)  [unwired: 1 in]
                    n2882 = Number To Decimal String(number=w5278) -> (decimal integer string=w5276:string)  [unwired: 1 in]
                    n2883 = Number To Decimal String(number=w5273) -> (decimal integer string=w5271:string)  [unwired: 1 in]
                    n2884 = Number To Fractional String(number=w5300, precision (6)=w5245) -> (F-format string=w5302:string)  [unwired: 2 in]
